vi "cDAQ Example.vi"(8 "Error In":errorcluster) -> (0 "Error Out":errorcluster)   [LabVIEW 2014]
doc: "Example that displays the components of the cDAQ. Shows how to initialize the cDAQ, acquire data, and close the cDAQ."
uses:
  Type Definitions/cDAQ Setup.ctl
  Type Definitions/Instrument Sensor.ctl
panel:
  out "AI Data":T1[](array[typedef])=[{"Mean"=0.23493816147116703, " Std"=0.26272546606576874, "Color Box"=6618880}, {"Mean"=0.010075320485673694, " Std"=0.0022149280740790594, "Color Box"=6618880}, {"Mean"=108.30275916239206, " Std"=0.0, "Color Box"=6618880}, {"Mean"=9.993391544228452, " Std"=0.00040217289696060823, "Color Box"=6618880}, {"Mean"=0.7762114319734401, " Std"=0.001631933671938549, "Color Box"=6618880}, {"Mean"=0.37705357820404206, " Std"=0.08873442057713618, "Color Box"=6618880}, {"Mean"=0.00746324710452399, " Std"=0.005433143618640284, "Color Box"=6618880}, {"Mean"=0.005952570103052505, " Std"=0.003834084808605862, "Color Box"=6618880}, {"Mean"=0.008711197664442945, " Std"=0.00823315758311951, "Color Box"=6618880}, {"Mean"=0.017249806797911993, " Std"=0.006526980769079336, "Color Box"=6618880}, {"Mean"=0.018103667714629415, " Std"=0.003777406352513851, "Color Box"=6618880}, {"Mean"=0.009433695370694195, " Std"=0.004950145332658338, "Color Box"=6618880}, {"Mean"=0.00378507700425324, " Std"=0.005371253875846873, "Color Box"=6618880}, {"Mean"=0.004179166653942727, " Std"=0.0069797333684830844, "Color Box"=6618880}, {"Mean"=0.007857336763257079, " Std"=0.0019092910491546487, "Color Box"=6618880}, {"Mean"=0.005492798843181003, " Std"=0.0015298316935691309, "Color Box"=6618880}, {"Mean"=0.002734171265893455, " Std"=0.0010742507769753928, "Color Box"=6618880}, {"Mean"=-0.00705238850632651, " Std"=0.0003284080469232783, "Color Box"=6618880}, {"Mean"=-0.001732178153977648, " Std"=0.0009112953439522598, "Color Box"=6618880}, {"Mean"=-0.010730558636110197, " Std"=0.001664870095149315, "Color Box"=6618880}, {"Mean"=-0.01992598399091939, " Std"=0.0010488511987790804, "Color Box"=6618880}, {"Mean"=-0.030106633545555577, " Std"=0.0017284374992287612, "Color Box"=6618880}]
  out "Temp Data":T1[](array[typedef])=[{"Mean"=-101440.14950293404, " Std"=5.658644743804699, "Color Box"=6618880}, {"Mean"=-101440.14950293404, " Std"=5.658644743804699, "Color Box"=6618880}, {"Mean"=-101440.14950293404, " Std"=5.658644743804699, "Color Box"=6618880}, {"Mean"=-101440.14950293404, " Std"=5.658644743804699, "Color Box"=6618880}, {"Mean"=-101440.14950293404, " Std"=5.658644743804699, "Color Box"=6618880}, {"Mean"=-101440.14950293404, " Std"=5.658644743804699, "Color Box"=6618880}, {"Mean"=-101440.14950293404, " Std"=5.658644743804699, "Color Box"=6618880}, {"Mean"=-101440.14950293404, " Std"=5.658644743804699, "Color Box"=6618880}, {"Mean"=71.75200545481124, " Std"=0.04486156319638956, "Color Box"=6618880}, {"Mean"=-101440.14950293404, " Std"=5.658644743804699, "Color Box"=6618880}, {"Mean"=-101440.14950293404, " Std"=5.658644743804699, "Color Box"=6618880}, {"Mean"=-101440.14950293404, " Std"=5.658644743804699, "Color Box"=6618880}, {"Mean"=-101440.14950293404, " Std"=5.658644743804699, "Color Box"=6618880}, {"Mean"=-101440.14950293404, " Std"=5.658644743804699, "Color Box"=6618880}, {"Mean"=-101440.14950293404, " Std"=5.658644743804699, "Color Box"=6618880}, {"Mean"=-101440.14950293404, " Std"=5.658644743804699, "Color Box"=6618880}, {"Mean"=-101479.57198271868, " Std"=12.632367099712763, "Color Box"=6618880}, {"Mean"=-101479.57198271868, " Std"=12.632367099712763, "Color Box"=6618880}, {"Mean"=-101479.57198271868, " Std"=12.632367099712763, "Color Box"=6618880}, {"Mean"=-101479.57198271868, " Std"=12.632367099712763, "Color Box"=6618880}, {"Mean"=-101479.57198271868, " Std"=12.632367099712763, "Color Box"=6618880}, {"Mean"=-101479.57198271868, " Std"=12.632367099712763, "Color Box"=6618880}, {"Mean"=-101479.57198271868, " Std"=12.632367099712763, "Color Box"=6618880}, {"Mean"=-101479.57198271868, " Std"=12.632367099712763, "Color Box"=6618880}, {"Mean"=-101479.57198271868, " Std"=12.632367099712763, "Color Box"=6618880}, {"Mean"=-101479.57198271868, " Std"=12.632367099712763, "Color Box"=6618880}, {"Mean"=-101479.57198271868, " Std"=12.632367099712763, "Color Box"=6618880}, {"Mean"=-101479.57198271868, " Std"=12.632367099712763, "Color Box"=6618880}, {"Mean"=-101479.57198271868, " Std"=12.632367099712763, "Color Box"=6618880}, {"Mean"=-101479.57198271868, " Std"=12.632367099712763, "Color Box"=6618880}, {"Mean"=-101479.57198271868, " Std"=12.632367099712763, "Color Box"=6618880}, {"Mean"=-101479.57198271868, " Std"=12.632367099712763, "Color Box"=6618880}, {"Mean"=-101399.74703674568, " Std"=10.627309799080603, "Color Box"=6618880}, {"Mean"=-101399.74703674568, " Std"=10.627309799080603, "Color Box"=6618880}, {"Mean"=-101399.74703674568, " Std"=10.627309799080603, "Color Box"=6618880}, {"Mean"=-101399.74703674568, " Std"=10.627309799080603, "Color Box"=6618880}, {"Mean"=-101399.74703674568, " Std"=10.627309799080603, "Color Box"=6618880}, {"Mean"=-101399.74703674568, " Std"=10.627309799080603, "Color Box"=6618880}, {"Mean"=-101399.74703674568, " Std"=10.627309799080603, "Color Box"=6618880}, {"Mean"=-101399.74703674568, " Std"=10.627309799080603, "Color Box"=6618880}, {"Mean"=-101399.74703674568, " Std"=10.627309799080603, "Color Box"=6618880}, {"Mean"=-101399.74703674568, " Std"=10.627309799080603, "Color Box"=6618880}, {"Mean"=-101399.74703674568, " Std"=10.627309799080603, "Color Box"=6618880}, {"Mean"=-101399.74703674568, " Std"=10.627309799080603, "Color Box"=6618880}, {"Mean"=-101399.74703674568, " Std"=10.627309799080603, "Color Box"=6618880}, {"Mean"=-101399.74703674568, " Std"=10.627309799080603, "Color Box"=6618880}, {"Mean"=-101399.74703674568, " Std"=10.627309799080603, "Color Box"=6618880}, {"Mean"=-101399.74703674568, " Std"=10.627309799080603, "Color Box"=6618880}, {"Mean"=-101405.06836384868, " Std"=13.607861565934025, "Color Box"=6618880}, {"Mean"=-101405.06836384868, " Std"=13.607861565934025, "Color Box"=6618880}, {"Mean"=-101405.06836384868, " Std"=13.607861565934025, "Color Box"=6618880}, {"Mean"=-101405.06836384868, " Std"=13.607861565934025, "Color Box"=6618880}, {"Mean"=-101405.06836384868, " Std"=13.607861565934025, "Color Box"=6618880}, {"Mean"=-101405.06836384868, " Std"=13.607861565934025, "Color Box"=6618880}, {"Mean"=-101405.06836384868, " Std"=13.607861565934025, "Color Box"=6618880}, {"Mean"=-101405.06836384868, " Std"=13.607861565934025, "Color Box"=6618880}, {"Mean"=-101405.06836384868, " Std"=13.607861565934025, "Color Box"=6618880}, {"Mean"=-101405.06836384868, " Std"=13.607861565934025, "Color Box"=6618880}, {"Mean"=-101405.06836384868, " Std"=13.607861565934025, "Color Box"=6618880}, {"Mean"=-101405.06836384868, " Std"=13.607861565934025, "Color Box"=6618880}, {"Mean"=-101405.06836384868, " Std"=13.607861565934025, "Color Box"=6618880}, {"Mean"=-101405.06836384868, " Std"=13.607861565934025, "Color Box"=6618880}, {"Mean"=-101405.06836384868, " Std"=13.607861565934025, "Color Box"=6618880}, {"Mean"=-101405.06836384868, " Std"=13.607861565934025, "Color Box"=6618880}, {"Mean"=76.23664254826167, " Std"=0.06183215576860884, "Color Box"=6618880}, {"Mean"=72.41647637494297, " Std"=0.152696079546221, "Color Box"=6618880}, {"Mean"=73.16835283891731, " Std"=0.17408230162122562, "Color Box"=6618880}, {"Mean"=73.45469643015343, " Std"=0.20827743903333404, "Color Box"=6618880}, {"Mean"=-101385.55439208687, " Std"=28.065396267120857, "Color Box"=6618880}, {"Mean"=-101385.55439208687, " Std"=28.065396267120857, "Color Box"=6618880}, {"Mean"=-101385.55439208687, " Std"=28.065396267120857, "Color Box"=6618880}, {"Mean"=-101385.55439208687, " Std"=28.065396267120857, "Color Box"=6618880}, {"Mean"=-101385.55439208687, " Std"=28.065396267120857, "Color Box"=6618880}, {"Mean"=-101385.55439208687, " Std"=28.065396267120857, "Color Box"=6618880}, {"Mean"=-101385.55439208687, " Std"=28.065396267120857, "Color Box"=6618880}, {"Mean"=-101385.55439208687, " Std"=28.065396267120857, "Color Box"=6618880}, {"Mean"=-101385.55439208687, " Std"=28.065396267120857, "Color Box"=6618880}, {"Mean"=-101385.55439208687, " Std"=28.065396267120857, "Color Box"=6618880}, {"Mean"=-101385.55439208687, " Std"=28.065396267120857, "Color Box"=6618880}, {"Mean"=-101385.55439208687, " Std"=28.065396267120857, "Color Box"=6618880}]
  out "cDAQ Data Out":dbl[](array[numeric])=[-101440.14950293404, 0.0, 0.0, 0.0, 0.0, 0.0, 0.0, 0.0, 0.0, 0.0, 0.0, 0.0, 0.0, 0.0, 0.0, 0.0, 0.0, 0.0, 0.0, 0.0, 0.0, 0.0, 0.0, 0.0, 0.0, 0.0, 0.0, 0.0, 0.0, 0.0, 0.0, 0.0, 0.0, 0.0, 0.0, 0.0, 0.0, 0.0, 0.0, 0.0, 0.0, 0.0, 0.0, 0.0, 0.0, 0.0, 0.0, 0.0, 0.0, 0.0, 0.0, 0.0, 0.0, 0.0, 0.0, 0.0, 0.0, 0.0, 0.0, 0.0, 0.0, 0.0, 0.0, 0.0, 0.0, 0.0, 0.0, 0.0, 0.0, 0.0, 0.0, 0.0, 0.0, 0.0, 0.0, 0.0, 0.0, 0.0, 0.0, 0.0, 0.0, 0.0, 0.0, 0.0, 0.0, 0.0, 0.0, 0.0, 0.0, 0.0, 0.0, 0.0, 0.0, 0.0, 0.0]
  in  "Setup":T2={"Test Setup"={"RH Resistor"=100.0, "Temp Resistor"=100.0, "Gas P. Resistor"=250.0, "Temp4mA Val"=32.0, "Temp20mA Val"=212.0, "RH4mA Val"=0.0, "RH20mA Val"=100.0, "GPres4mA Val"=0.0, "Gpres20mA Val"=50.0}, "cDAQ Array Locations"={"Scale Channel"=90, "TC Channels"=0, "VDC Discrete Channel"=72, "RH Chan"=91, "Temp Chan"=93, "Tscale Channel"=2, "RDB Channel"=0, "Gas Temperature"=88, "Gas Pressure"=89, "Barometric Pressure"=94, "Gas Feedback Chan"=92}}
  in  "DAQmx Task (Analog Input Volt)":refnum<k21>="AI Voltage"
  in  "DAQmx Task (Temperature)":refnum<k21>="Temperature"
  in  "stop":bool
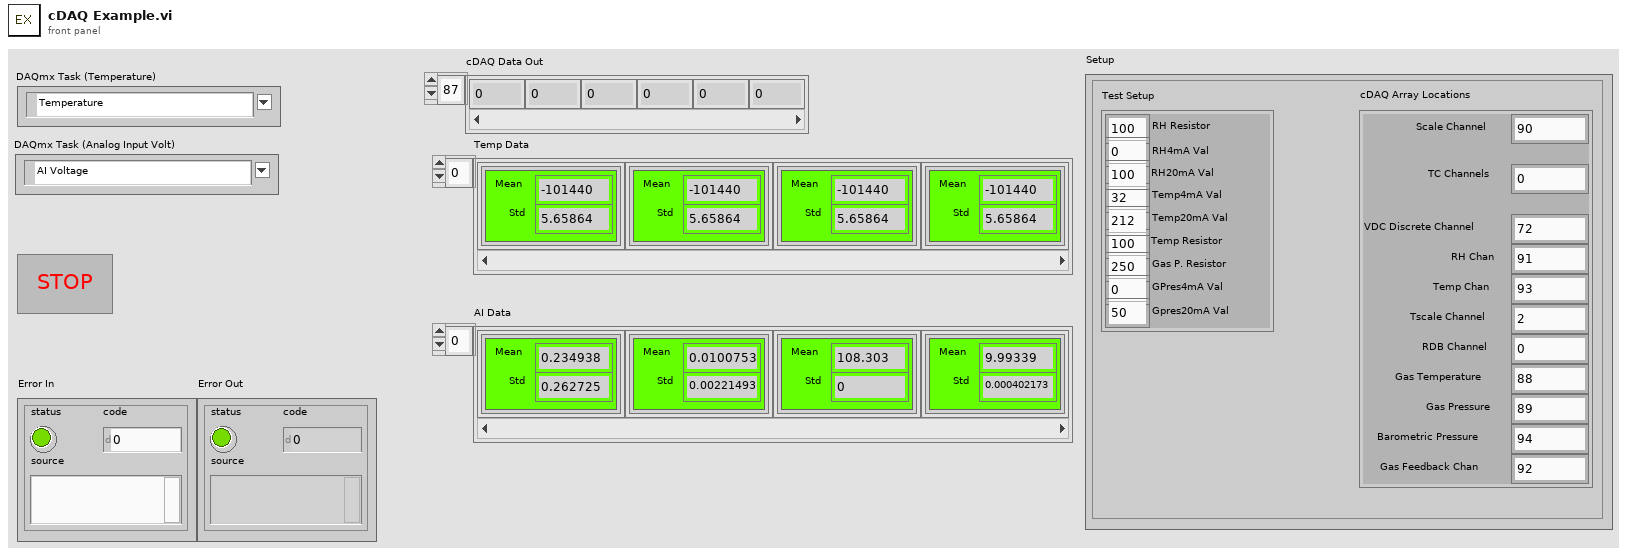
[diagram p1: front panel]
types:
  T1 = typedef "Instrument Sensor.ctl" = cluster{"Mean":dbl, " Std":dbl, "Color Box":u32}
  T2 = typedef "cDAQ Setup.ctl" = cluster{"Test Setup":cluster{"RH Resistor":dbl, "Temp Resistor":dbl, "Gas P. Resistor":dbl, "Temp4mA Val":dbl, "Temp20mA Val":dbl, "RH4mA Val":dbl, "RH20mA Val":dbl, "GPres4mA Val":dbl, "Gpres20mA Val":dbl}, "cDAQ Array Locations":cluster{"Scale Channel":i32, "TC Channels":i32, "VDC Discrete Channel":i32, "RH Chan":i32, "Temp Chan":i32, "Tscale Channel":i32, "RDB Channel":i32, "Gas Temperature":i32, "Gas Pressure":i32, "Barometric Pressure":i32, "Gas Feedback Chan":i32}}
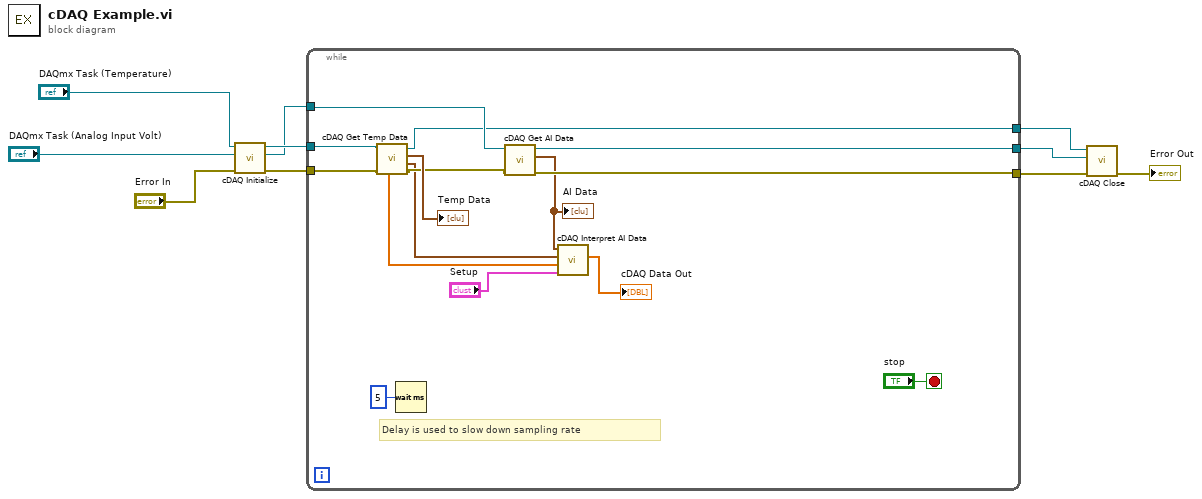
[diagram p0: block diagram]
diagram:
  n1 = call "cDAQ Initialize.vi"("DAQmx Task (Temperature)"="DAQmx Task (Temperature)", "DAQmx Task (Analog Input Volt)"="DAQmx Task (Analog Input Volt)", "Error In"="Error In") -> ("Temp Task Out"=w4:refnum<k21>, "AI Task Out"=w3:refnum<k21>, "Error Out"=w9:errorcluster)  [unwired: 5 in]
  n2 = while {
    tunnel: w9 -> [w18]
    tunnel: [w22] -> w8
    tunnel: w4 -> [w17]
    tunnel: w3 -> [w21]
    tunnel: [w20] -> w2
    tunnel: [w16] -> w1
    stop <- "stop" stop-if-true
    # "Delay is used to slow down sampling rate"
    n3 = call "cDAQ Get Temp Data.vi"("Error In"=w18, "Input Task"=w17) -> ("Error Out"=w13:errorcluster, "Gas Temp"=w12:T1, "Mean & StdDev"=→"Temp Data":T1[], "Task Out"=w16:refnum<k21>, "to cDAQ output"=w14:dbl[])  [unwired: 3 in, 1 out]
    n4 = Wait (ms)(milliseconds to wait=u32 5) -> ()  [unwired: 1 out]
    n5 = call "cDAQ Get AI Data.vi"("Error In"=w13, "Input Task"=w21) -> ("Error Out"=w22:errorcluster, "Mean & StdDev"=w19:T1[], "Task Out"=w20:refnum<k21>)  [unwired: 6 in, 1 out]
    "AI Data" <- w19
    n6 = call "cDAQ Interpret AI Data.vi"("AI Data"=w19, "Gas Temp"=w12, "Temp Means"=w14, "Setup"="Setup") -> ("cDAQ Data Out"=→"cDAQ Data Out":dbl[])  [unwired: 6 in]
  }
  n7 = call "cDAQ Close.vi"("Error In"=w8, "AI Task"=w2, "Temp Task"=w1) -> ("Error Out"=→"Error Out":errorcluster)  [unwired: 8 in]
